vi "LIA_7230_setup.vi"(3 "error in (no error)":errorcluster, 4 "VISA  session":refnum<visa-resource-name>, 5 "LIA7230-Settings":T1={"Interface"=1, "Port"=0, "Serial Number"="08199244", "IP Address"="192.168.11.6", "Line Frequency\nRejection Filter"=0, "Input Mode"=1, "Input Conn. Shells"=TRUE, "Line Frequency"=FALSE, "Auto AC Gain"=FALSE, "AC Gain"=0, "Input Device"=FALSE, "Range"=26, " Auto Sensitivity "=FALSE, "Auto Measure"=FALSE, "Range 2"=25, " Auto Sensitivity  2"=FALSE, "Slope"=1, "Synchronous TC"=FALSE, "Time Constant"=12, "Slope 2"=1, "Time Constant 2"=12, "Oscillator Amp (V rms)"=0.5, "Oscillator Freq (Hz)"=150000.0, "Reference I/P"=0, "Ref Harm 1"=1, "Ref Harm2"=2, "Virtual Ref.\nMode"=FALSE, "Dual Harmonic/Reference Mode"=FALSE, "Reference Mode"=FALSE, "TRIG OUT\n= Ref Mon"=FALSE, " Auto Phase "=FALSE, "Reference Phase 1"=0.0, "+90 degrees 1"=FALSE, " Auto Phase 2 "=FALSE, "Reference 2 Phase"=0.0, "+90 degrees2"=FALSE, "Auxiliary I/O"=FALSE, "Configuration"=FALSE, "Curve Buffer"=FALSE, "Offsets"=FALSE, "X Channel Offset (%)"=-6.7055225e-06, "X Channel Offset"=FALSE, "Y Channel Offset (%)"=-6.705522537231445e-06, "Y Channel Offset"=FALSE, " Auto Offset"=FALSE, "X Channel Offset (%) 2"=-6.7055225e-06, "X Channel Offset 2"=FALSE, "Y Channel Offset (%) 2"=-6.705522537231445e-06, "Y Channel Offset 2"=FALSE, " Auto Offset 2"=FALSE, "Display Type channel 1"=5, "Display Type channel 2"=5, "Display Type channel 3"=5, "Display Type channel 4"=5, "Osc Sweeps"=FALSE, "Define Equation1"=FALSE, "Coupling"=FALSE} {"Display Type channel 4" items=["X %", "Y %", "X Calibrated", "Y Calibrated", "Mag %", "Mag Calibrated", "Phase Degrees", "Ratio", "Log Ratio", "ADC 1", "ADC 2", "ADC 3", "ADC 4", "Noise %", "Noise Calibrated", "Ref Frequency", "Equation 1", "Equation 2", "X2 %", "Y2 %", "X2 Calibrated", "Y2 Calibrated", "Mag2 %", "Mag2 Calibrated", "Phase2 Degrees"]; "Display Type channel 3" items=["X %", "Y %", "X Calibrated", "Y Calibrated", "Mag %", "Mag Calibrated", "Phase Degrees", "Ratio", "Log Ratio", "ADC 1", "ADC 2", "ADC 3", "ADC 4", "Noise %", "Noise Calibrated", "Ref Frequency", "Equation 1", "Equation 2", "X2 %", "Y2 %", "X2 Calibrated", "Y2 Calibrated", "Mag2 %", "Mag2 Calibrated", "Phase2 Degrees"]; "Display Type channel 2" items=["X %", "Y %", "X Calibrated", "Y Calibrated", "Mag %", "Mag Calibrated", "Phase Degrees", "Ratio", "Log Ratio", "ADC 1", "ADC 2", "ADC 3", "ADC 4", "Noise %", "Noise Calibrated", "Ref Frequency", "Equation 1", "Equation 2", "X2 %", "Y2 %", "Mag2 %", "Mag2 Calibrated", "Phase2 Degrees"]; "Display Type channel 1" items=["X %", "Y %", "X Calibrated", "Y Calibrated", "Mag %", "Mag Calibrated", "Phase Degrees", "Ratio", "Log Ratio", "ADC 1", "ADC 2", "ADC 3", "ADC 4", "Noise %", "Noise Calibrated", "Ref Frequency", "Equation 1", "Equation 2", "X2 %", "Y2 %", "Mag2 %", "Mag2 Calibrated", "Phase2 Degrees"]; "Y Channel Offset (%) 2" format="%.2f"; "X Channel Offset (%) 2" min=-300 max=300 step=0.01 format="%.2f"; "Y Channel Offset (%)" format="%.2f"; "X Channel Offset (%)" min=-300 max=300 step=0.01 format="%.2f"; "Reference 2 Phase" min=-200.0 max=200.0 step=0.01 scale=-180.0..180.0 scale format="%.1f"; "Reference Phase 1" min=-200.0 max=200.0 step=0.01 scale=-180.0..180.0 scale format="%.1f"; "Ref Harm2" min=1 max=127 step=1; "Ref Harm 1" min=1 max=127 step=1; "Reference I/P" items=["Internal", "External TTL (Rear Panel)", "External (Front Panel)"]; "Oscillator Freq (Hz)" min=0.5 max=150000.0 step=0.001 format="%.3f"; "Oscillator Amp (V rms)" min=0.0 max=5.0 step=0.0001 format="%.3f"; "Time Constant 2" items=["10µs", "20µs", "50µs", "100µs", "200µs", "500µs", "1ms", "2ms", "5ms", "10ms", "20ms", "50ms", "100ms", "200ms", "500ms", "1s", "2s", "5s", "10s", "20s", "50s", "100s", "200s", "500s", "1ks", "2ks", "5ks", "10ks", "20ks", "50ks", "100ks"]; "Slope 2" items=["6db/octave", "12dB/octave", "18dB/octave", "24dB/octave"]; "Time Constant" items=["10µs", "20µs", "50µs", "100µs", "200µs", "500µs", "1ms", "2ms", "5ms", "10ms", "20ms", "50ms", "100ms", "200ms", "500ms", "1s", "2s", "5s", "10s", "20s", "50s", "100s", "200s", "500s", "1ks", "2ks", "5ks", "10ks", "20ks", "50ks", "100ks"]; "Slope" items=["6db/octave", "12dB/octave", "18dB/octave", "24dB/octave"]; "Range 2" items=["N/A", "2nV", "5nV", "10nV", "20nV", "50nV", "100nV", "200nV", "500nV", "1µV", "2µV", "5µV", "10µV", "20µV", "50µV", "100µV", "200µV", "500µV", "1mV", "2mV", "5mV", "10mV", "20mV", "50mV", "100mV", "200mV", "500mV", "1V"]; "Range" items=["N/A", "2nV", "5nV", "10nV", "20nV", "50nV", "100nV", "200nV", "500nV", "1µV", "2µV", "5µV", "10µV", "20µV", "50µV", "100µV", "200µV", "500µV", "1mV", "2mV", "5mV", "10mV", "20mV", "50mV", "100mV", "200mV", "500mV", "1V"]; "AC Gain" items=["0dB", "6dB", "12dB", "18dB", "24dB", "30dB", "36dB", "42dB", "48dB", "54dB", "60dB", "66dB", "78dB", "84dB", "90dB"]; "Input Mode" items=["Inputs Grounded (test)", "A (Single-Ended Voltage)", "-B (Inverting Single Ended Voltage)", "A-B (Differential Voltage)", "AUX Input - Main Console", "B Current input - Wide Bandwidth", "B Current input - Low Noise"]; "Line Frequency\nRejection Filter" items=["OFF", "F", "2F", "F & 2F"]; "Port" items=["COM 1", "COM 2", "COM 3", "COM 4", "COM 5", "COM 6", "COM 7", "COM 8", "COM 9", "COM 10"]; "Interface" items=["RS232", "USB", "Ethernet"]}) -> (0 "error out":errorcluster, 1 "Offsets (ON)":bool, 2 "Visa session (out)":refnum<visa-resource-name>)   [LabVIEW 2019]
uses:
  Monitor Communication/LIA7230/Settings_cluster.ctl
  Equipment/LIA7230/SR7230LV8.llb/SR7230 VISA Write/Read.vi
panel:
  # "USB Interface"
  # "Ethernet Interface"
  # "Oscillator"
  # "Output Channels -Offset"
  # "Reference Control"
  # "Dual Reference/\nDual Harmonic"
  # "Single Reference/\nSingle Harmonic"
  # "Dual"
  # "Input Configuration"
  # "Output Channels TC & Slope"
  # "Single"
  # "On"
  # "On"
  # "Single mode"
  # "Dual mode"
  # "Off"
  # "Off"
  # "DC"
  # "Dual Ref. Mode"
  # "AC"
  # "Dual Harm. Mode"
  # "On"
  # "On"
  # "Off"
  # "Off"
  # "On"
  # "Float"
  # "On"
  # "On"
  # "Off"
  # "Ground"
  # "Off"
  # "Off"
  # "FET"
  # "Sensitivity"
  # "50 Hz"
  # "On"
  # "Dual mode"
  # "Single mode"
  # "Bipolar"
  # "60 Hz"
  # "Off"
  # "Degrees"
  # "Degrees"
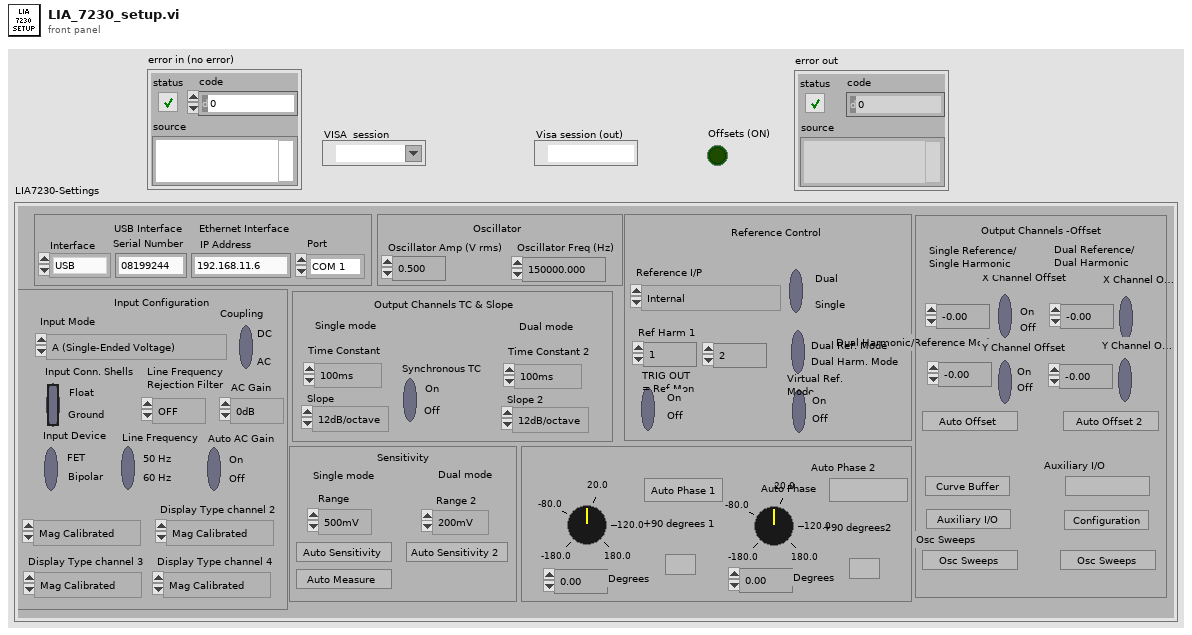
[diagram p1: front panel]
types:
  T1 = typedef "Settings_cluster.ctl" = cluster{"Interface":u16, "Port":u16, "Serial Number":string, "IP Address":string, "Line Frequency\nRejection Filter":u8, "Input Mode":u16, "Input Conn. Shells":bool, "Line Frequency":bool, "Auto AC Gain":bool, "AC Gain":u16, "Input Device":bool, "Range":u8, " Auto Sensitivity ":bool, "Auto Measure":bool, "Range 2":u8, " Auto Sensitivity  2":bool, "Slope":u8, "Synchronous TC":bool, "Time Constant":u16, "Slope 2":u8, "Time Constant 2":u16, "Oscillator Amp (V rms)":dbl, "Oscillator Freq (Hz)":dbl, "Reference I/P":u8, "Ref Harm 1":u16, "Ref Harm2":u16, "Virtual Ref.\nMode":bool, "Dual Harmonic/Reference Mode":bool, "Reference Mode":bool, "TRIG OUT\n= Ref Mon":bool, " Auto Phase ":bool, "Reference Phase 1":dbl, "+90 degrees 1":bool, " Auto Phase 2 ":bool, "Reference 2 Phase":dbl, "+90 degrees2":bool, "Auxiliary I/O":bool, "Configuration":bool, "Curve Buffer":bool, "Offsets":bool, "X Channel Offset (%)":sgl, "X Channel Offset":bool, "Y Channel Offset (%)":dbl, "Y Channel Offset":bool, " Auto Offset":bool, "X Channel Offset (%) 2":sgl, "X Channel Offset 2":bool, "Y Channel Offset (%) 2":dbl, "Y Channel Offset 2":bool, " Auto Offset 2":bool, "Display Type channel 1":u16, "Display Type channel 2":u16, "Display Type channel 3":u16, "Display Type channel 4":u16, "Osc Sweeps":bool, "Define Equation1":bool, "Coupling":bool}
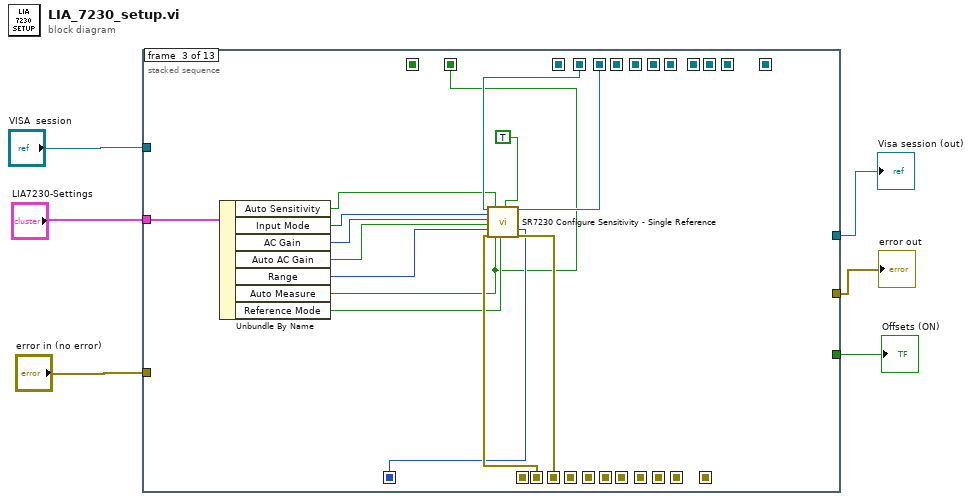
[diagram p0: block diagram]
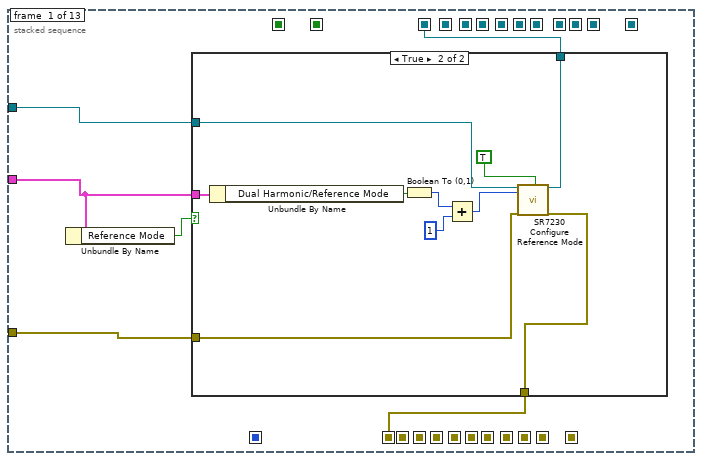
[diagram p2: hidden frame]
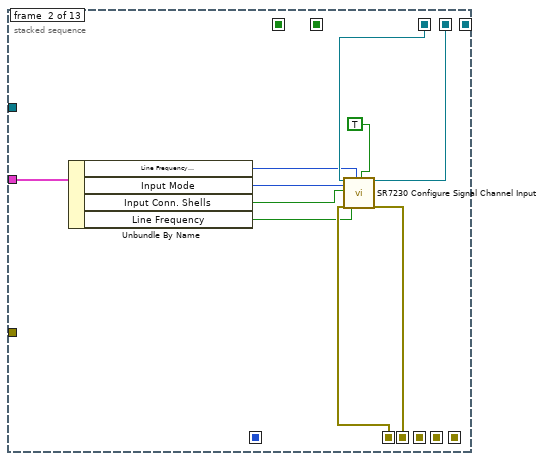
[diagram p4: hidden frame]
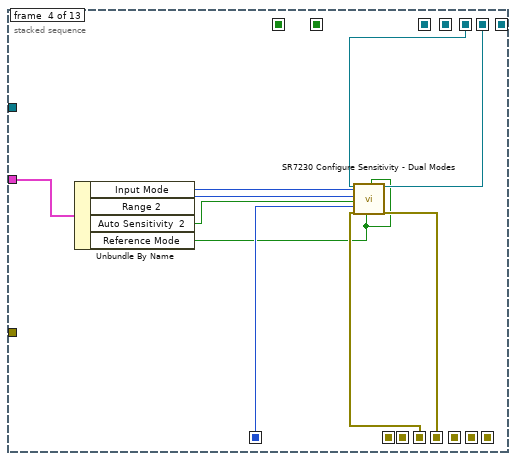
[diagram p5: hidden frame]
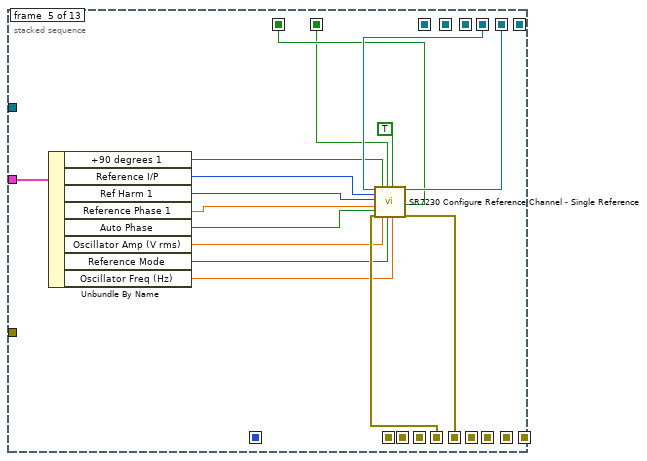
[diagram p6: hidden frame]
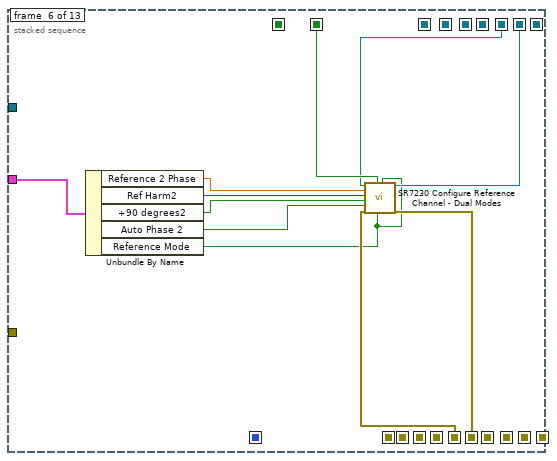
[diagram p7: hidden frame]
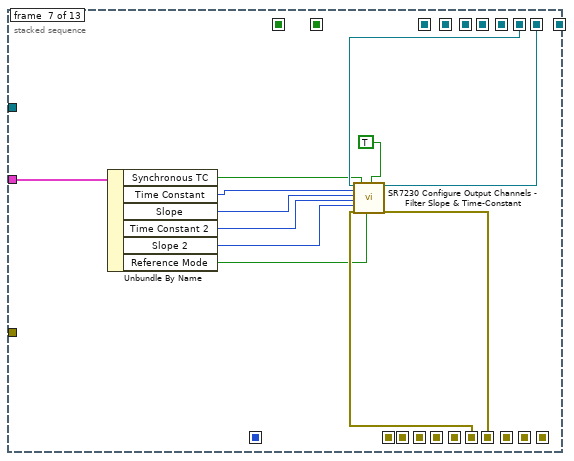
[diagram p8: hidden frame]
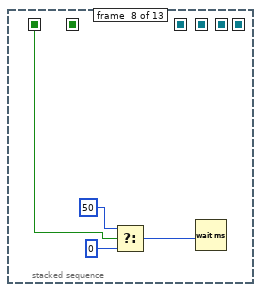
[diagram p9: hidden frame]
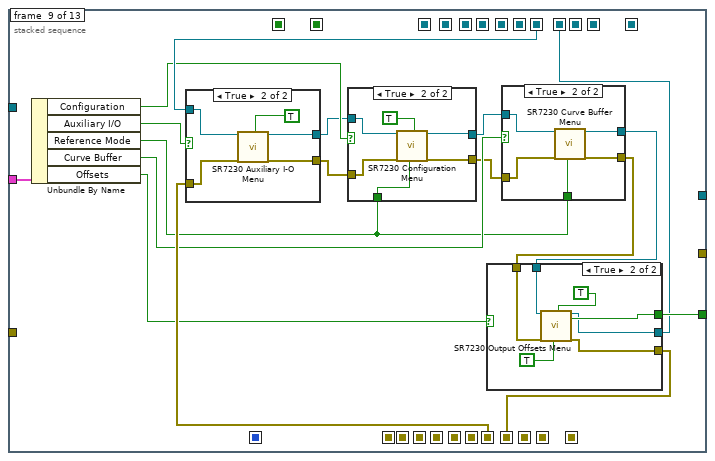
[diagram p10: hidden frame]
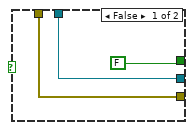
[diagram p11: hidden frame]
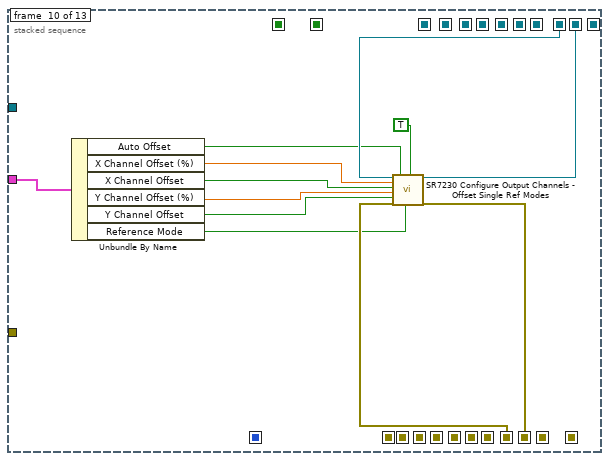
[diagram p15: hidden frame]
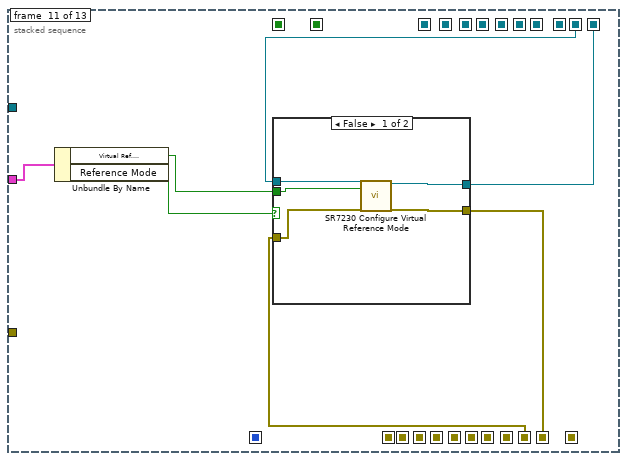
[diagram p16: hidden frame]
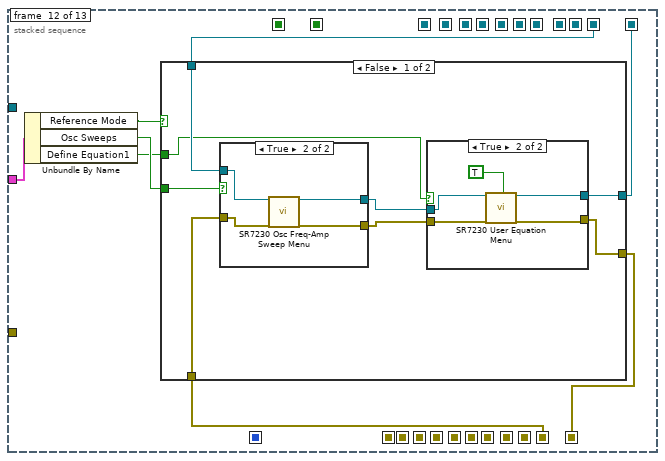
[diagram p18: hidden frame]
diagram:
  n1 = stacked-sequence {
    seq-local: [w12 _ _ _ _ _ _ _ _ _ _ _ _] -> [_ w31 _ _ _ _ _ _ _ _ _ _ _]
    seq-local: [w11 _ _ _ _ _ _ _ _ _ _ _ _] -> [_ w33 _ _ _ _ _ _ _ _ _ _ _]
    seq-local: [_ w32 _ _ _ _ _ _ _ _ _ _ _] -> [_ _ w39 _ _ _ _ _ _ _ _ _ _]
    seq-local: [_ w30 _ _ _ _ _ _ _ _ _ _ _] -> [_ _ w47 _ _ _ _ _ _ _ _ _ _]
    seq-local: [_ _ w46 _ _ _ _ _ _ _ _ _ _] -> [_ _ _ w58 _ _ _ _ _ _ _ _ _]
    seq-local: [_ _ w38 _ _ _ _ _ _ _ _ _ _] -> [_ _ _ w56 _ _ _ _ _ _ _ _ _]
    seq-local: [_ _ _ w57 _ _ _ _ _ _ _ _ _] -> [_ _ _ _ w74 _ _ _ _ _ _ _ _]
    seq-local: [_ _ _ w55 _ _ _ _ _ _ _ _ _] -> [_ _ _ _ w72 _ _ _ _ _ _ _ _]
    seq-local: [_ _ w36 _ _ _ _ _ _ _ _ _ _] -> [_ _ _ w50 _ _ _ _ _ _ _ _ _]
    seq-local: [_ _ _ _ w73 _ _ _ _ _ _ _ _] -> [_ _ _ _ _ w80 _ _ _ _ _ _ _]
    seq-local: [_ _ _ _ w71 _ _ _ _ _ _ _ _] -> [_ _ _ _ _ w85 _ _ _ _ _ _ _]
    seq-local: [_ _ _ _ w62 _ _ _ _ _ _ _ _] -> [_ _ _ _ _ _ _ w98 _ _ _ _ _]
    seq-local: [_ _ w35 _ _ _ _ _ _ _ _ _ _] -> [_ _ _ _ w60 w82 _ _ _ _ _ _ _]
    seq-local: [_ _ _ _ _ w83 _ _ _ _ _ _ _] -> [_ _ _ _ _ _ w95 _ _ _ _ _ _]
    seq-local: [_ _ _ _ _ w84 _ _ _ _ _ _ _] -> [_ _ _ _ _ _ w93 _ _ _ _ _ _]
    seq-local: [_ _ _ _ _ _ w94 _ _ _ _ _ _] -> [_ _ _ _ _ _ _ _ w118 _ _ _ _]
    seq-local: [_ _ _ _ _ _ w92 _ _ _ _ _ _] -> [_ _ _ _ _ _ _ _ w117 _ _ _ _]
    seq-local: [_ _ _ _ _ _ _ _ w103 _ _ _ _] -> [_ _ _ _ _ _ _ _ _ w162 _ _ _]
    seq-local: [_ _ _ _ _ _ _ _ w102 _ _ _ _] -> [_ _ _ _ _ _ _ _ _ w161 _ _ _]
    seq-local: [_ _ _ _ _ _ _ _ _ w152 _ _ _] -> [_ _ _ _ _ _ _ _ _ _ w167 _ _]
    seq-local: [_ _ _ _ _ _ _ _ _ w151 _ _ _] -> [_ _ _ _ _ _ _ _ _ _ w166 _ _]
    seq-local: [_ _ _ _ _ _ _ _ _ _ w164 _ _] -> [_ _ _ _ _ _ _ _ _ _ _ w181 _]
    seq-local: [_ _ _ _ _ _ _ _ _ _ w163 _ _] -> [_ _ _ _ _ _ _ _ _ _ _ w180 _]
    seq-local: [_ _ _ _ _ _ _ _ _ _ _ w178 _] -> [_ _ _ _ _ _ _ _ _ _ _ _ w210]
    seq-local: [_ _ _ _ _ _ _ _ _ _ _ w177 _] -> [_ _ _ _ _ _ _ _ _ _ _ _ w211]
    tunnel: "LIA7230-Settings" -> [w8 w34 w48 w54 w70 w81 w96 _ w116 w160 w169 w184 w215]
    tunnel: "VISA  session" -> [w10 _ _ _ _ _ _ _ _ _ _ _ _]
    tunnel: "error in (no error)" -> [w9 _ _ _ _ _ _ _ _ _ _ _ _]
    tunnel: [_ _ _ _ _ _ _ _ w106 _ _ _ _] -> w3
    tunnel: [_ _ _ _ _ _ _ _ _ _ _ _ w209] -> w2
    tunnel: [_ _ _ _ _ _ _ _ _ _ _ _ w208] -> w1
    frame #0 {
      n2 = Unbundle By Name(w8) -> ("Reference Mode"=w7:bool)
      n3 = case shown="True" w7 {
        tunnel: [w14 w23] -> w12
        tunnel: [w13 w22] -> w11
        tunnel: w10 -> [w14 w21]
        tunnel: w8 -> [_ w20]
        tunnel: w9 -> [w13 w19]
        frame False {
        }
        frame True {
          n4 = Unbundle By Name(w20) -> ("Dual Harmonic/Reference Mode"=w18:bool)
          n5 = Boolean To (0,1)(Boolean=w18) -> (0, 1=w17:i16)
          n6 = Add(x=w17, y=1) -> (x+y=w16:i32)
          n7 = call "SR7230 Configure Reference Mode.vi"("VISA session (for class)"=w21, "Reference Channel Mode"=w16, "error in (no error)"=w19, "Update"=TRUE) -> ("dup VISA session"=w23:refnum<visa-resource-name>, "error out"=w22:errorcluster)  [unwired: 14 in]
        }
      }
    }
    frame #1 {
      n8 = Unbundle By Name(w34) -> ("Line Frequency\nRejection Filter"=w26:u8, "Input Mode"=w27:u16, "Input Conn. Shells"=w28:bool, "Line Frequency"=w29:bool)
      n9 = call "SR7230 Configure Signal Channel Input.vi"("VISA session (for class)"=w31, "Input Mode"=w27, "Input Connector Shells"=w28, "error in (no error)"=w33, "Line Frequency"=w29, "Line Frequency\nRejection Filter"=w26, "Update"=TRUE) -> ("VISA session"=w30:refnum<visa-resource-name>, "error out"=w32:errorcluster)  [unwired: 10 in, 1 out]
    }
    frame #2 {
      n10 = Unbundle By Name(w48) -> ("Auto Sensitivity"=w44:bool, "Input Mode"=w43:u16, "AC Gain"=w42:u16, "Auto AC Gain"=w41:bool, "Range"=w40:u8, "Auto Measure"=w35:bool, "Reference Mode"=w37:bool)
      n11 = call "SR7230 Configure Sensitivity - Single Reference.vi"("VISA session (for class)"=w47, "Input Mode"=w43, "AC Gain"=w42, "Auto AC Gain"=w41, "Range"=w40, "error in (no error)"=w39, "Auto Sensitivity"=w44, "Auto Measure"=w35, "Reference Mode"=w37, "Update"=TRUE) -> ("VISA session"=w46:refnum<visa-resource-name>, "ACGAIN out"=w36:i32, "error out"=w38:errorcluster)  [unwired: 3 in, 4 out]
    }
    frame #3 {
      n12 = Unbundle By Name(w54) -> ("Input Mode"=w53:u16, "Range 2"=w52:u8, "Auto Sensitivity  2"=w51:bool, "Reference Mode"=w49:bool)
      n13 = call "SR7230 Configure Sensitivity - Dual Modes.vi"("VISA session (for class)"=w58, "Input Mode"=w53, "Range 2"=w52, "Auto Sensitivity 2"=w51, "AC Gain In"=w50, "error in (no error)"=w56, "Reference Mode"=w49, "Update"=w49) -> ("dup VISA session"=w57:refnum<visa-resource-name>, "error out"=w55:errorcluster)  [unwired: 6 in, 4 out]
    }
    frame #4 {
      n14 = Unbundle By Name(w70) -> ("+90 degrees 1"=w59:bool, "Reference I/P"=w69:u8, "Ref Harm 1"=w68:u16, "Reference Phase 1"=w67:dbl, "Auto Phase"=w66:bool, "Oscillator Amp (V rms)"=w65:dbl, "Reference Mode"=w64:bool, "Oscillator Freq (Hz)"=w63:dbl)
      n15 = call "SR7230 Configure Reference Channel - Single Reference.vi"("VISA session (for class)"=w74, "Reference Input"=w69, "Reference\nHarmonic"=w68, "Reference Phase"=w67, "Auto Phase"=w66, "error in (no error)"=w72, "+90 degrees"=w59, "Oscillator Amp (V rms)"=w65, "Update Reference Phase"=w60, "Reference Mode"=w64, "Update"=TRUE, "Oscillator Freq (Hz)"=w63) -> ("VISA session"=w73:refnum<visa-resource-name>, "Ref Locked"=w62:bool, "error out"=w71:errorcluster)  [unwired: 1 in, 4 out]
    }
    frame #5 {
      n16 = Unbundle By Name(w81) -> ("Reference 2 Phase"=w79:dbl, "Ref Harm2"=w78:u16, "+90 degrees2"=w77:bool, "Auto Phase 2"=w76:bool, "Reference Mode"=w75:bool)
      n17 = call "SR7230 Configure Reference Channel - Dual Modes.vi"("VISA session (for class)"=w80, "Reference Phase"=w79, "Reference\nHarmonic 2"=w78, "+90 degrees"=w77, "Auto Phase"=w76, "error in (no error)"=w85, "Update Reference Phase"=w82, "Reference Mode"=w75, "Update"=w75) -> ("VISA session"=w83:refnum<visa-resource-name>, "error out"=w84:errorcluster)  [unwired: 6 in, 3 out]
    }
    frame #6 {
      n18 = Unbundle By Name(w96) -> ("Synchronous TC"=w91:bool, "Time Constant"=w90:u16, "Slope"=w89:u8, "Time Constant 2"=w88:u16, "Slope 2"=w87:u8, "Reference Mode"=w86:bool)
      n19 = call "SR7230 Configure Output Channels - Filter Slope & Time-Constant.vi"("VISA session (for class)"=w95, "Time Constant"=w90, "Slope"=w89, "Time Constant 2"=w88, "Slope 2"=w87, "error in (no error)"=w93, "Synchronous TC"=w91, "Reference Mode"=w86, "Update"=TRUE) -> ("VISA session"=w94:refnum<visa-resource-name>, "error out"=w92:errorcluster)  [unwired: 4 in, 5 out]
    }
    frame #7 {
      n20 = Select(t=50, s=w98, f=0) -> (s? t:f=w101:i32)
      n21 = Wait (ms)(milliseconds to wait=w101) -> ()  [unwired: 1 out]
    }
    frame #8 {
      n22 = Unbundle By Name(w116) -> ("Configuration"=w114:bool, "Auxiliary I/O"=w115:bool, "Reference Mode"=w108:bool, "Curve Buffer"=w111:bool, "Offsets"=w107:bool)
      n23 = case shown="True" w115 {
        tunnel: w118 -> [w145 w150]
        tunnel: w117 -> [w144 w149]
        tunnel: [w145 w147] -> w113
        tunnel: [w144 w146] -> w112
        frame False {
        }
        frame True {
          n24 = call "SR7230 Auxiliary I-O Menu.vi"("VISA session (for class)"=w150, "error in (no error)"=w149, "Update"=TRUE) -> ("dup VISA session"=w147:refnum<visa-resource-name>, "error out"=w146:errorcluster)  [unwired: 15 in]
        }
      }
      n25 = case shown="True" w114 {
        tunnel: w113 -> [w137 w143]
        tunnel: w112 -> [w136 w142]
        tunnel: w108 -> [_ w140]
        tunnel: [w137 w139] -> w110
        tunnel: [w136 w138] -> w109
        frame False {
        }
        frame True {
          n26 = call "SR7230 Configuration Menu.vi"("VISA session (for class)"=w143, "error in (no error)"=w142, "Refmode"=w140, "Update"=TRUE) -> ("dup VISA session"=w139:refnum<visa-resource-name>, "error out"=w138:errorcluster)  [unwired: 14 in]
        }
      }
      n27 = case shown="True" w111 {
        tunnel: w110 -> [w130 w135]
        tunnel: w109 -> [w129 w134]
        tunnel: w108 -> [_ w133]
        tunnel: [w130 w132] -> w105
        tunnel: [w129 w131] -> w104
        frame False {
        }
        frame True {
          n28 = call "SR7230 Curve Buffer Menu.vi"("VISA session (for class)"=w135, "error in (no error)"=w134, "Reference Mode"=w133) -> ("dup VISA session"=w132:refnum<visa-resource-name>, "error out"=w131:errorcluster)  [unwired: 15 in]
        }
      }
      n29 = case shown="True" w107 {
        tunnel: [FALSE w127] -> w106
        tunnel: w105 -> [w120 w126]
        tunnel: w104 -> [w119 w125]
        tunnel: [w120 w123] -> w103
        tunnel: [w119 w122] -> w102
        frame False {
        }
        frame True {
          n30 = call "SR7230 Output Offsets Menu.vi"("VISA session (for class)"=w126, "error in (no error)"=w125, "Reference Mode"=TRUE, "Update"=TRUE) -> ("dup VISA session"=w123:refnum<visa-resource-name>, "Offset(s) ON"=w127:bool, "error out"=w122:errorcluster)  [unwired: 13 in]
        }
      }
    }
    frame #9 {
      n31 = Unbundle By Name(w160) -> ("Auto Offset"=w154:bool, "X Channel Offset (%)"=w159:sgl, "X Channel Offset"=w158:bool, "Y Channel Offset (%)"=w157:dbl, "Y Channel Offset"=w156:bool, "Reference Mode"=w155:bool)
      n32 = call "SR7230 Configure Output Channels - Offset Single Ref Modes.vi"("VISA session (for class)"=w162, "X Channel Offset (%)"=w159, "X Channel Offset"=w158, "Y Channel Offset (%)"=w157, "Y Channel Offset"=w156, "error in (no error)"=w161, "Auto Offset"=w154, "Ref Mode"=w155, "Update"=TRUE) -> ("VISA session"=w152:refnum<visa-resource-name>, "error out"=w151:errorcluster)  [unwired: 4 in, 5 out]
    }
    frame #10 {
      n33 = Unbundle By Name(w169) -> ("Virtual Ref.\nMode"=w165:bool, "Reference Mode"=w168:bool)
      n34 = case shown="False" w168 {
        tunnel: w167 -> [w174 w176]
        tunnel: w166 -> [w173 w175]
        tunnel: [w172 w176] -> w164
        tunnel: [w171 w175] -> w163
        tunnel: w165 -> [w170 _]
        frame False {
          n35 = call "SR7230 Configure Virtual Reference Mode.vi"("VISA session (for class)"=w174, "Virtual Reference\nMode"=w170, "error in (no error)"=w173) -> ("VISA session"=w172:refnum<visa-resource-name>, "error out"=w171:errorcluster)  [unwired: 15 in]
        }
        frame True {
        }
      }
    }
    frame #11 {
      n36 = Unbundle By Name(w184) -> ("Reference Mode"=w183:bool, "Osc Sweeps"=w182:bool, "Define Equation1"=w179:bool)
      n37 = case shown="False" w183 {
        tunnel: w182 -> [w192 _]
        tunnel: w181 -> [w191 w207]
        tunnel: w180 -> [w190 w206]
        tunnel: w179 -> [w189 _]
        tunnel: [w186 w207] -> w177
        tunnel: [w185 w206] -> w178
        frame False {
          n38 = case shown="True" w192 {
            tunnel: w191 -> [w201 w205]
            tunnel: w190 -> [w200 w204]
            tunnel: [w201 w203] -> w188
            tunnel: [w200 w202] -> w187
            frame False {
            }
            frame True {
              n39 = call "SR7230 Osc Freq-Amp Sweep Menu.vi"("VISA session (for class)"=w205, "error in (no error)"=w204) -> ("dup VISA session"=w203:refnum<visa-resource-name>, "error out"=w202:errorcluster)  [unwired: 16 in]
            }
          }
          n40 = case shown="True" w189 {
            tunnel: w188 -> [w194 w199]
            tunnel: w187 -> [w193 w198]
            tunnel: [w194 w196] -> w186
            tunnel: [w193 w195] -> w185
            frame False {
            }
            frame True {
              n41 = call "SR7230 User Equation Menu.vi"("VISA session (for class)"=w199, "error in (no error)"=w198, "Update"=TRUE) -> ("dup VISA session"=w196:refnum<visa-resource-name>, "error out"=w195:errorcluster)  [unwired: 15 in]
            }
          }
        }
        frame True {
        }
      }
    }
    frame #12 {
      n42 = Unbundle By Name(w215) -> ("Coupling"=w212:bool)
      n43 = Format Into String(format string="DCCOUPLE %d", w212) -> (resulting string=w213:string)  [unwired: 2 in, 1 out]
      n44 = call "SR7230 VISA Write/Read.vi"("VISA session (for class)"=w211, "Write Command String"=w213, "error in (no error)"=w210) -> ("VISA session"=w209:refnum<visa-resource-name>, "error out"=w208:errorcluster)  [unwired: 4 in, 11 out]
    }
  }
  "error out" <- w1
  "Offsets (ON)" <- w3
  "Visa session (out)" <- w2
